vi "PWM Init.vi"(5 "Phase-Correct (F)":bool, 7 "GPIO #":T1=-1, 8 "error in (no error)":errorcluster, 10 "Enable (F)":bool, 11 "VisaComms in":refnum<class "VisaComms.lvclass">) -> (0 "error out":errorcluster, 3 "VisaComms out":refnum<class "VisaComms.lvclass">)   [LabVIEW 2020, in "CTI.lvlib" / "VisaComms.lvclass"]
uses:
  VisaComms.lvclass
  GPIO Number.ctl
  VisaComms.lvclass/VisaComms.ctl
  CTI.lvlib
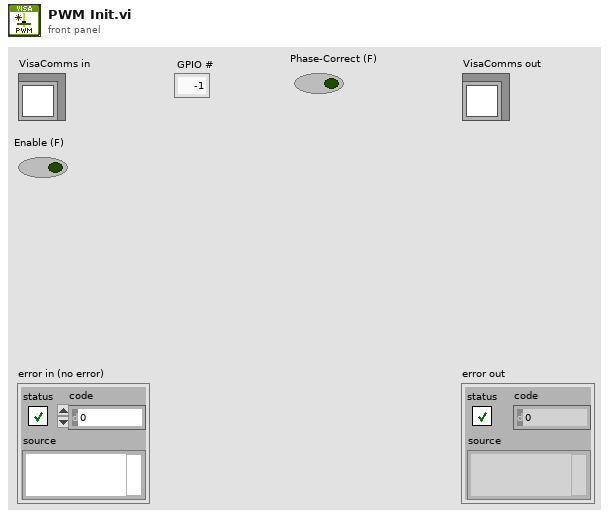
[diagram p1: front panel]
types:
  T1 = typedef "CTI.lvlib/GPIO Number.ctl" = i8
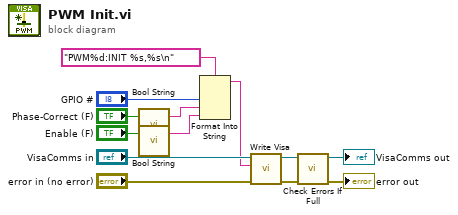
[diagram p0: block diagram]
diagram:
  n1 = call "Bool String.vi"("Bool"="Phase-Correct (F)") -> ("String"=w8:string)  [unwired: 6 in]
  n2 = call "Bool String.vi"("Bool"="Enable (F)") -> ("String"=w7:string)  [unwired: 6 in]
  n3 = Format Into String(format string="PWM%d:INIT %s,%s\n", "GPIO #", w8, w7) -> (resulting string=w4:string)  [unwired: 2 in, 1 out]
  n4 = call "Write Visa.vi"("error in (no error)"="error in (no error)", "write buffer"=w4, "VisaComms in"="VisaComms in") -> ("error out"=w6:errorcluster, "VisaComms out"=w2:refnum<class "VisaComms.lvclass">)  [unwired: 6 in, 1 out]
  n5 = call "Check Errors If Full.vi"("error in (no error)"=w6, "VisaComms in"=w2) -> ("error out"=→"error out":errorcluster, "VisaComms out"=→"VisaComms out":refnum<class "VisaComms.lvclass">)  [unwired: 8 in]
